vi "Set All Channels.vi"(8 "error in":errorcluster, 10 "Channels[]":refnum<class "Plugin_Channels.lvclass">[](array[class]), 11 "Module Configuration in":refnum<class "Module Configuration.lvclass">) -> (0 "error out":errorcluster, 3 "Module Configuration out":refnum<class "Module Configuration.lvclass">)   [LabVIEW 2020, in "Plugin.lvlib" / "Plugin_UI.lvclass"]
doc: "Enabled channels are written to module configuration, and output channel's scale settings is disabled."
uses:
  Plugin_UI.lvclass
  builds/Libraries/LabSys Framework.lvlibp/Configuration Storage/Module Configuration/Module Configuration.lvclass
  Channels/Plugin_Channels.lvclass
  builds/Libraries/LabSys Framework.lvlibp/Configuration Storage/Test Configuration/Channel Directions.ctl
  builds/Libraries/Shared GUI Library.lvlibp/Shared GUI Library/Scale Settings Dialog/Scale Settings Dialog.lvlib
  builds/Libraries/LabSys Framework.lvlibp/Configuration Storage/Test Configuration/Test Configuration.lvclass
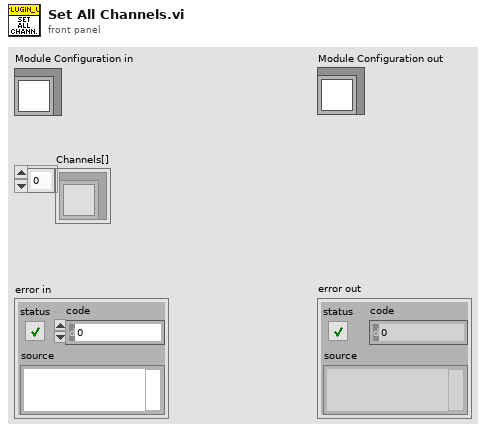
[diagram p1: front panel]
types:
  T1 = typedef "LabSys Framework.lvlibp/Configuration Storage.lvlib/Test Configuration.lvclass/Channel Directions.ctl" = enum8{"Module Input", "Module Output"}
  T2 = typedef "LabSys Framework.lvlibp/Configuration Storage.lvlib/Test Configuration.lvclass/Channel Information.ctl" = cluster{"Channel Direction":T1, "Alias":string, "Refresh (ms)":dbl, "Scaling Information":T3, "Value Type":T5, "Subchannels":T6[], "Auxiliary Data":variant}
  T3 = typedef "LabSys Framework.lvlibp/Configuration Storage.lvlib/Test Configuration.lvclass/Scaling Information.ctl" = cluster{"Active":bool, "Scaling Type":T4, "Output Minimum":dbl, "Output Maximum":dbl, "Raw Minimum":dbl, "Raw Maximum":dbl, "Output Unit":string, "Function":string, "Lookup Table":string}
  T4 = typedef "LabSys Framework.lvlibp/Configuration Storage.lvlib/Test Configuration.lvclass/Scaling Types.ctl" = enum8{"Linear", "Function", "Lookup Table"}
  T5 = typedef "Framework Base Library.lvlibp/Value Types.ctl" = enum8{"Unknown", "double", "double array", "Waveform", "DigWaveform", "Boolean", "Decimal", "String", "Db2Message", "Byte Array", "Unsigned Decimal"}
  T6 = typedef "LabSys Framework.lvlibp/Configuration Storage.lvlib/Test Configuration.lvclass/Subchannel Information.ctl" = cluster{"Alias":string, "Start Bit":u32, "Bit Length":u32, "Value Type":T5, "Auxiliary Data":variant}
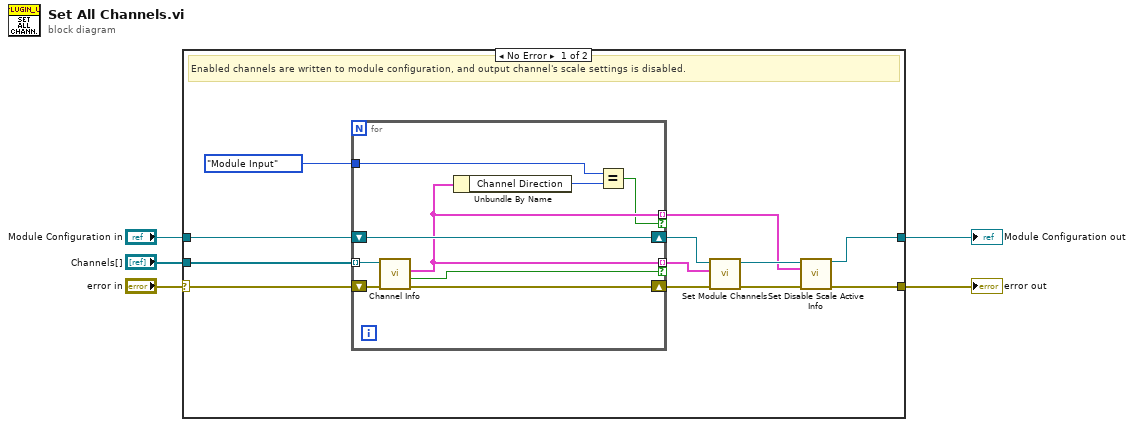
[diagram p0: block diagram]
diagram:
  n1 = case shown="No Error" "error in" {
    selector: "error in" -> [w17 w28]
    tunnel: [w9 w28] -> w4
    tunnel: "Module Configuration in" -> [w13 w27]
    tunnel: [w7 w27] -> w2
    tunnel: "Channels[]" -> [w15 _]
    frame No Error {
      # "Enabled channels are written to module configuration, and output channel's scale settings is disabled."
      n2 = for {
        tunnel: w15 -> [w25] mode=indexing
        shift-right: [w24] -> w16
        shift-left: w17 -> [w26]
        tunnel: [w19] -> w14 mode=indexing if=w22
        shift-right: [w23] -> w12
        shift-left: w13 -> [w23]
        tunnel: Channel_Directions."Module Input" ("x") -> [w20]
        tunnel: [w19] -> w6 mode=indexing if=w18
        n3 = call-dynamic "Channel Info.vi"("error in"=w26, "Plugin_Channels in"=w25) -> ("error out"=w24:errorcluster, "Channel Active?"=w22:bool, "Channel Information"=w19:T2)  [unwired: 6 in, 1 out]
        n4 = Unbundle By Name(w19) -> ("Channel Direction"=w21:T1)
        n5 = Equal?(x=w20, y=w21) -> (x = y?=w18:bool)
      }
      n6 = call-dynamic "Set Module Channels.vi"("error in (no error)"=w16, "Channel Information"=w14, "Module Configuration in"=w12) -> ("error out"=w10:errorcluster, "Module Configuration out"=w8:refnum<class "Module Configuration.lvclass">)  [unwired: 7 in]
      n7 = call "Set Disable Scale Active Info.vi"("Module Configuration in"=w8, "ChannelInfo"=w6, "error in (no error)"=w10) -> ("Module Configuration out"=w7:refnum<class "Module Configuration.lvclass">, "error out"=w9:errorcluster)  [unwired: 11 in]
    }
    frame Error {
    }
  }
  "error out" <- w4
  "Module Configuration out" <- w2
